vi "exp_读取.vi"(2 "命令":string, 3 "帧数":i32=2) -> (0 "error out":errorcluster, 1 "数组":string[](array[string]))   [LabVIEW 2014]
panel:
  out "读到的帧数":dbl
  in  "目标IP":string="192.168.0.2"
  in  "最大值(548)":i32=1024
  out "Actual Receive Buffer Size":u32
  in  "Set Receive Buffer Size(byte)":u32=64000000
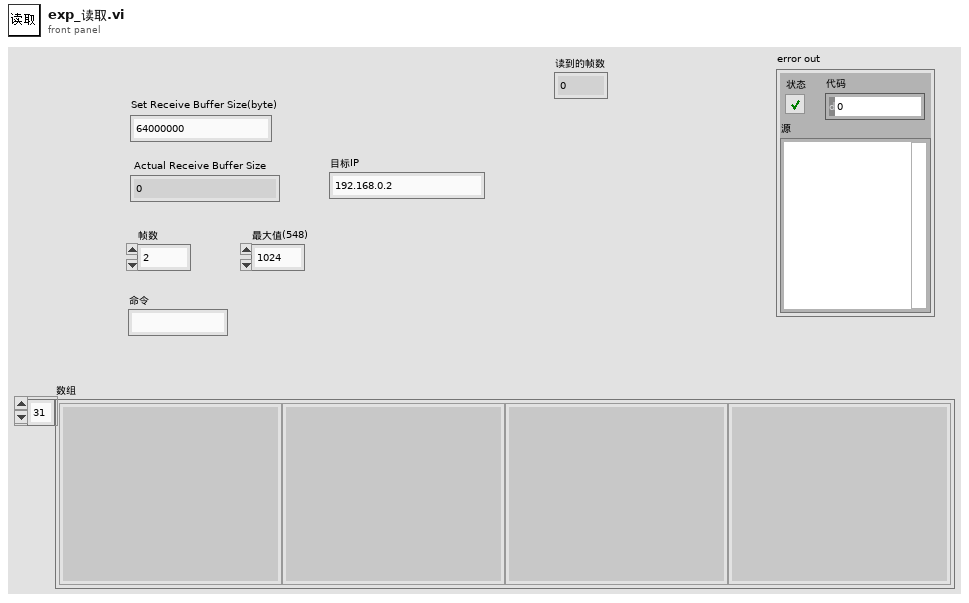
[diagram p1: front panel]
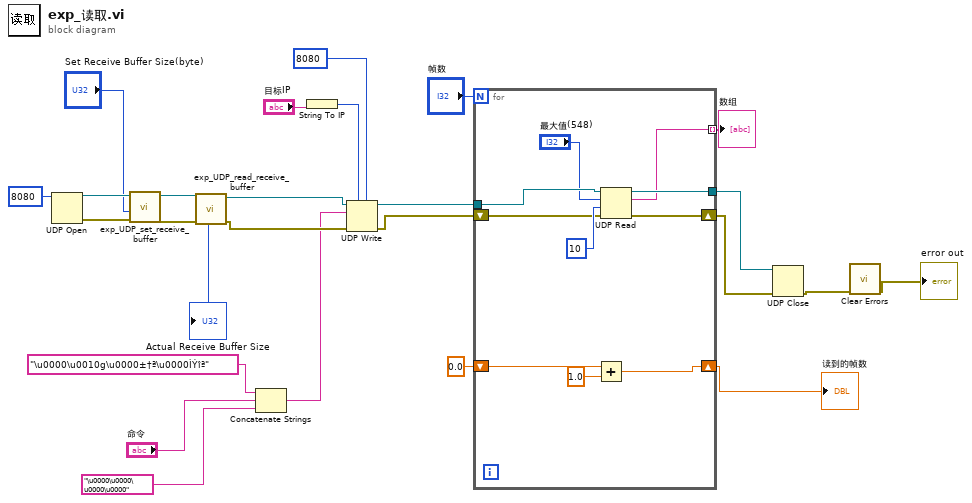
[diagram p0: block diagram]
diagram:
  n1 = UDP Open(11:u16 8080 ("端口")) -> (port=w23:refnum<k16>, 0:w22:errorcluster)  [unwired: 4 in, 1 out]
  n2 = call "exp_UDP_set_receive_buffer.vi"("error in (no error)"=w22, "Receive Buffer Size"="Set Receive Buffer Size(byte)", "connection ID"=w23) -> ("error out"=w20:errorcluster, "connection ID out"=w21:refnum<k16>)  [unwired: 6 in]
  n3 = call "exp_UDP_read_receive_buffer.vi"("error in (no error)"=w20, "connection ID"=w21) -> ("error out"=w17:errorcluster, "Receive Buffer Size"=→"Actual Receive Buffer Size":u32, "connection ID out"=w18:refnum<k16>)  [unwired: 5 in]
  n4 = Concatenate Strings("\u0000\u0010g\u0000±†ª\u0000ÌÝîª" ("字符串"), "命令", "\u0000\u0000\u0000\u0000" ("字符串")) -> (w8:string)
  n5 = String To IP(1:"目标IP") -> (0:w25:u32)
  n6 = UDP Write(address=w25, port or service name=u16 8080 ("端口或服务名称"), connection ID=w18, data in=w8, 8:w17) -> (error out=w15:errorcluster, 3:w16:refnum<k16>)  [unwired: 1 in]
  n7 = for {
    N: "帧数" -> [_]
    tunnel: w16 -> [w35]
    tunnel: [w33] -> w13
    tunnel: [w32] -> w11 mode=indexing
    shift-right: [w30] -> w9
    shift-left: w15 -> [w34]
    shift-right: [w27] -> w3
    shift-left: 0.0 -> [w28]
    n8 = Add(x=w28, y=1.0) -> (x+y=w27:dbl)
    n9 = UDP Read(connection ID=w35, max size (548)="最大值(548)", timeout ms (25000)=10 ("超时毫秒(25000)"), 8:w34) -> (data out=w32:string, error out=w30:errorcluster, 3:w33:refnum<k16>)  [unwired: 2 out]
  }
  "数组" <- w11
  "读到的帧数" <- w3
  n10 = UDP Close(connection ID=w13, 8:w9) -> (error out=w2:errorcluster)  [unwired: 1 out]
  n11 = call <vilib>:"Clear Errors.vi"("error in (no error)"=w2) -> ("error out"=→"error out":errorcluster)  [unwired: 5 in, 1 out]
